vi "Data Sheet.vi"(0 "Table":string[][](table), 2 "Page Header":cluster{"TITLE":string}={"TITLE"="TEST DATA SHEET (1 of 1)\nAPS3200 APU "}) -> ()   [LabVIEW 2018]
doc: "This is page 1 of the 36-300 data sheet"
panel:
  # "CHANNEL"
  # "MEASUREMENT"
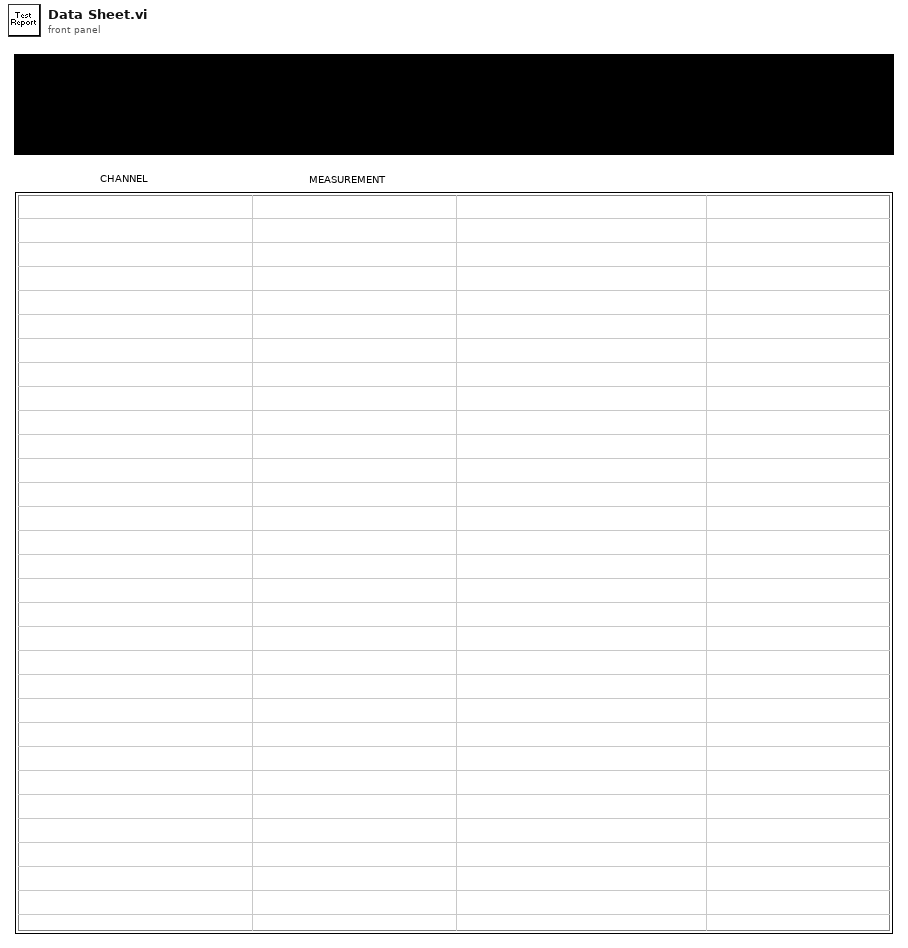
[diagram p1: front panel]
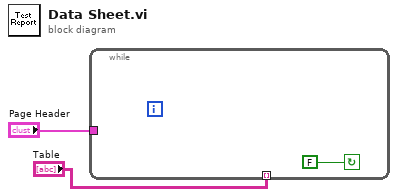
[diagram p0: block diagram]
diagram:
  n1 = while {
    tunnel: "Page Header" -> [_]
    tunnel: "Table" -> [_] mode=indexing
    stop <- FALSE continue-if-true
  }
